vi "Stamp tester.vi"() -> ()   [LabVIEW 2010]
uses:
  Stamp/Stamp 2 control.ctl
  Peristaltic/Pump w direction.ctl
  Stamp/mini peristaltic pump.ctl
  Stamp/Pump Direction.ctl
  Stamp/3-stop colors and numbers.ctl
  Stamp/stamp command.ctl
panel:
  out "error out":errorcluster
  in  "stop":bool
  out "success?":bool
  in  "Pump Number":u16 max=5 step=1
  in  "Pump":T3 {"0 to 1" min=0.0 max=1.0 step=0.01 scale=0.0..1.0 scale format="%.2g"}
  in  "Solenoids":bool[](array[boolean])
  in  "Control":T4={"Switches"=[FALSE, FALSE, FALSE], "Pumps"=[{"on/off"=FALSE, "Direction"=FALSE, "flow rate"=0.0, "Tubing"=enum."orange-black", "tubing or 0 to 1"=FALSE, "0 to 1"=0.0}, {"on/off"=FALSE, "Direction"=FALSE, "flow rate"=0.0, "Tubing"=enum."orange-black", "tubing or 0 to 1"=FALSE, "0 to 1"=0.0}, {"on/off"=FALSE, "Direction"=FALSE, "flow rate"=0.0, "Tubing"=enum."orange-black", "tubing or 0 to 1"=FALSE, "0 to 1"=0.0}, {"on/off"=FALSE, "Direction"=FALSE, "flow rate"=0.0, "Tubing"=enum."orange-black", "tubing or 0 to 1"=FALSE, "0 to 1"=0.0}, {"on/off"=FALSE, "Direction"=FALSE, "flow rate"=0.0, "Tubing"=enum."orange-black", "tubing or 0 to 1"=FALSE, "0 to 1"=0.0}, {"on/off"=FALSE, "Direction"=FALSE, "flow rate"=0.0, "Tubing"=enum."orange-black", "tubing or 0 to 1"=FALSE, "0 to 1"=0.0}]} {"Pumps"."0 to 1" format="%.2f"; "Pumps"."flow rate" format="%.2f"}
  in  "Serial Port":refnum<visa-resource-name>
  # "0-12"
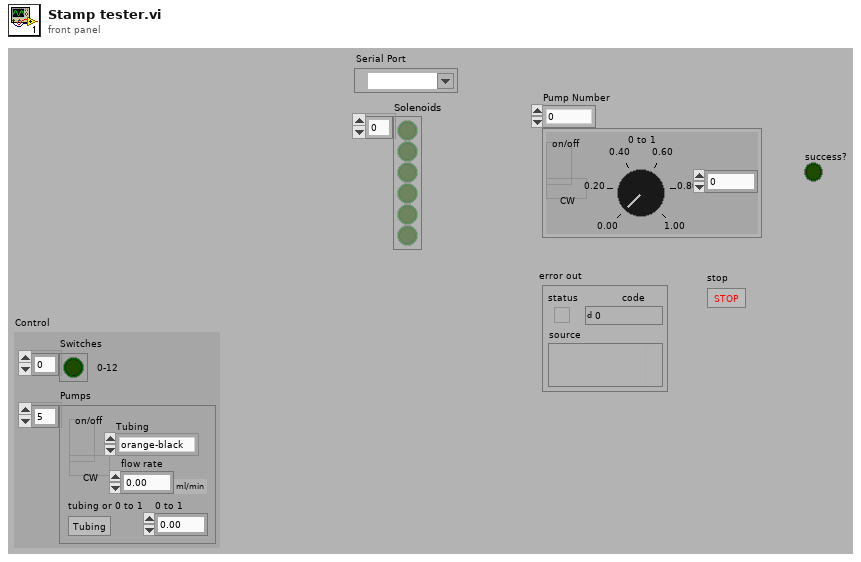
[diagram p1: front panel]
types:
  T1 = typedef "mini peristaltic pump.ctl" = bool
  T2 = typedef "Pump Direction.ctl" = bool
  T3 = cluster{"on/off":T1, "Direction":T2, "0 to 1":dbl}
  T4 = typedef "Stamp 2 control.ctl" = cluster{"Switches":bool[], "Pumps":T5[]}
  T5 = typedef "Pump w direction.ctl" = cluster{"on/off":T1, "Direction":T2, "flow rate":dbl[unit], "Tubing":T6, "tubing or 0 to 1":bool, "0 to 1":dbl}
  T6 = typedef "3-stop colors and numbers.ctl" = enum16{"orange-black", "orange-red", "orange-blue", "orange-green", "green-yellow", "orange-yellow", "white-yellow", "orange-white", "black-black", "orange-orange", "white-black", "white-white", "white-red", "red-red", "red-grey", "grey-grey", "yellow-yellow", "yellow-blue", "blue-blue", "blue-green", "green-green", "purple-purple", "purple-black", "purple-orange", "purple-white", "black-white", "13", "14", "15", "16", "17", "18"}
  T7 = typedef "stamp command.ctl" = enum16{"Configure", "Write", "Off", "Close"}
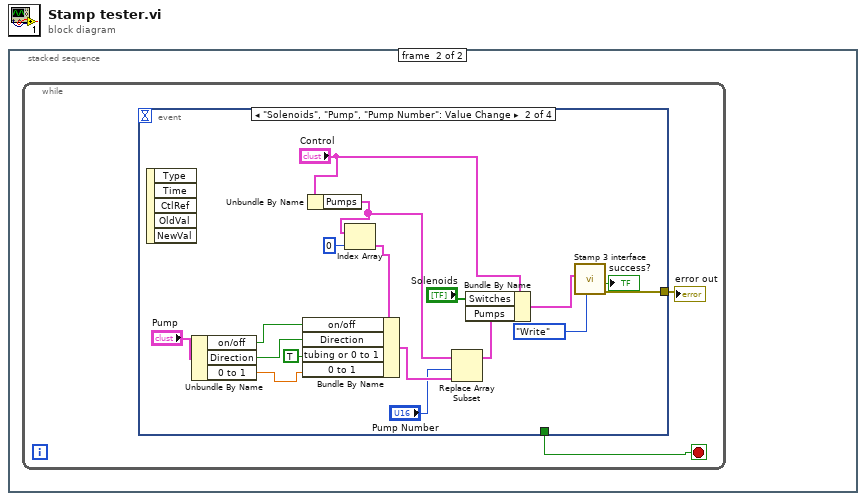
[diagram p0: block diagram]
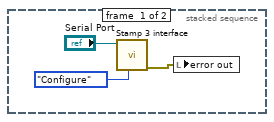
[diagram p2: hidden frame]
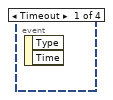
[diagram p3: hidden frame]
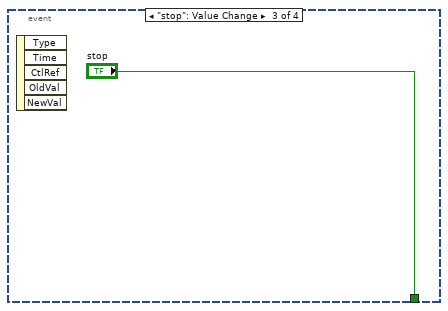
[diagram p4: hidden frame]
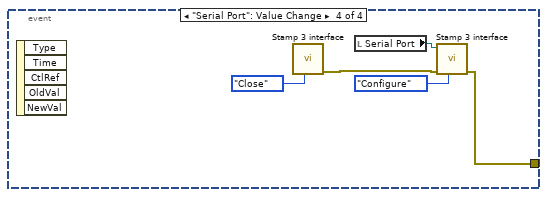
[diagram p5: hidden frame]
diagram:
  n1 = stacked-sequence {
    frame #0 {
      n2 = call "Stamp 3 interface.vi"("Stamp Command"=stamp_command."Configure", "Serial Port"="Serial Port") -> ("error out"=w1:errorcluster)  [unwired: 7 in, 2 out]
      n3 = local write "error out"(w1) -> ()
    }
    frame #1 {
      n4 = while {
        stop <- w5 stop-if-true
        n5 = event shown="[1] \"Solenoids\", \"Pump\", \"Pump Number\": Value Change" {
          selector: _ -> [_ _ _ _]
          dyn-events: _ -> [_ _ _ _]
          timeout: _ -> [_ _ _ _]
          tunnel: [_ _ "stop" _] -> w5
          tunnel: [_ w6 _ w24] -> w4
          event Timeout {
            n6 = event-data() -> ()  [unwired: 1 in, 2 out]
          }
          event "Solenoids", "Pump", "Pump Number": Value Change {
            n7 = event-data() -> ()  [unwired: 1 in, 5 out]
            n8 = Unbundle By Name("Pump") -> ("on/off"=w18:T1, "Direction"=w17:T2, "0 to 1"=w16:dbl)
            n9 = Unbundle By Name("Control") -> ("Pumps"=w15:T5[])
            n10 = Index Array(array=w15, index=0) -> (element=w21:T5)
            n11 = Bundle By Name(cluster=w21, "on/off"=w18, "Direction"=w17, "tubing or 0 to 1"=TRUE, "0 to 1"=w16) -> (w14:T5)
            n12 = Replace Array Subset(array=w15, new element=w14, index="Pump Number") -> (w12:T5[])
            n13 = Bundle By Name(cluster="Control", "Switches"="Solenoids", "Pumps"=w12) -> (w10:T4)
            n14 = call "Stamp 3 interface.vi"("Stamp Command"=stamp_command."Write", "Control"=w10) -> ("error out"=w6:errorcluster, "success?"=→"success?":bool)  [unwired: 7 in, 1 out]
          }
          event "stop": Value Change {
            n15 = event-data() -> ()  [unwired: 1 in, 5 out]
          }
          event "Serial Port": Value Change {
            n16 = event-data() -> ()  [unwired: 1 in, 5 out]
            n17 = call "Stamp 3 interface.vi"("Stamp Command"=stamp_command."Close") -> ("error out"=w26:errorcluster)  [unwired: 8 in, 2 out]
            n18 = local read "Serial Port"() -> (w25:refnum<visa-resource-name>)
            n19 = call "Stamp 3 interface.vi"("Stamp Command"=stamp_command."Configure", "error in (no error)"=w26, "Serial Port"=w25) -> ("error out"=w24:errorcluster)  [unwired: 6 in, 2 out]
          }
        }
        "error out" <- w4
      }
    }
  }
